vi "save operation binary.vi"(8 "error in":errorcluster, 11 "state cluster":T1) -> (0 "error out":errorcluster, 3 "state out":T1)   [LabVIEW 2013, in "RT Temperature Controller.lvlib"]
uses:
  RT Temperature Controller.lvlib
  Controls/StateCluster.ctl
  <vilib>/NI/Tag Bus Data Framework/Configuration Editor/Classes/SystemConfigRepo/SystemConfigRepo.lvclass
  <vilib>/CEF_TreeControl/Node/NodeRef.ctl
  <vilib>/CEF_TreeControl/Node/NISE_CEF_Node.lvclass
  <vilib>/CEF_TreeControl/Node/UserEventRef.ctl
  <vilib>/CEF_TreeControl/Controls/EventCluster.ctl
  SplashScreen/splash screen.ctl
  SplashScreen/notifier data.ctl
  <vilib>/NI/Tag Bus Data Framework/Configuration Editor/Classes/SystemConfigRepo/SystemConfigRepo.lvclass/SystemConfigRepo.ctl
  <vilib>/CEF_TreeControl/NISE_CEF_TreeControl.lvlib
  SplashScreen/splash screen.lvlib
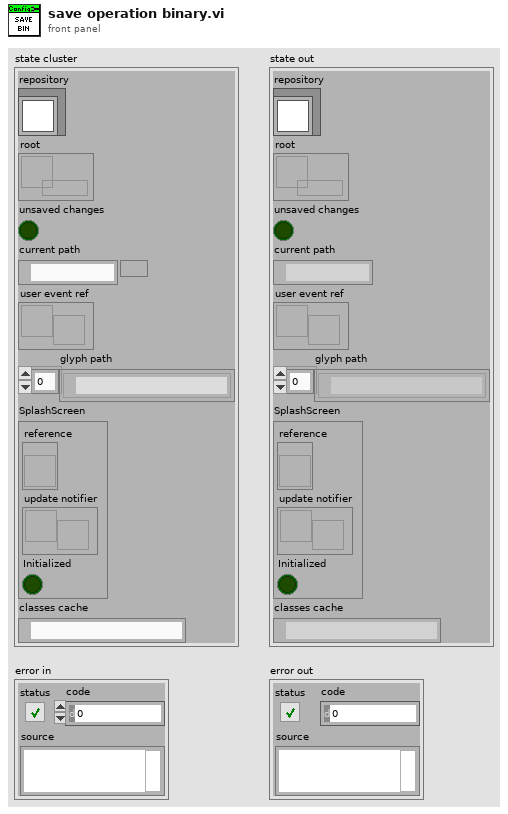
[diagram p1: front panel]
types:
  T1 = typedef "RT Temperature Controller.lvlib/StateCluster.ctl" = cluster{"repository":refnum<class "SystemConfigRepo.lvclass">, "root":T2, "unsaved changes":bool, "current path":path, "user event ref":T3, "glyph path":path[], "SplashScreen":T4, "classes cache":path}
  T2 = typedef "NISE_CEF_Node.lvclass/NodeRef.ctl" = refnum<data-value>
  T3 = typedef "NISE_CEF_Node.lvclass/UserEventRef.ctl" = refnum<user-event>
  T4 = typedef "RT Temperature Controller.lvlib/splash screen.lvlib/splash screen.ctl" = cluster{"reference":refnum<vi>, "update notifier":refnum<notifier>, "Initialized":bool}
  T5 = enum16{"open", "replace", "create", "open or create", "replace or create", "replace or create with confirmation"}
  T6 = typedef "PLConfigurationSerializer.lvlib/systems cluster.ctl" = cluster{"System Configuration":refnum<class "PL_System Configuration.lvclass">, "targets":T7[]}
  T7 = typedef "PLConfigurationSerializer.lvlib/targets cluster.ctl" = cluster{"Target Configuration":refnum<class "PL_Target Configuration.lvclass">, "engines":T8[]}
  T8 = typedef "PLConfigurationSerializer.lvlib/engines cluster.ctl" = cluster{"engine configuration":refnum<class "engine configuration.lvclass">, "modules":refnum<class "TBM module configuration.lvclass">[]}
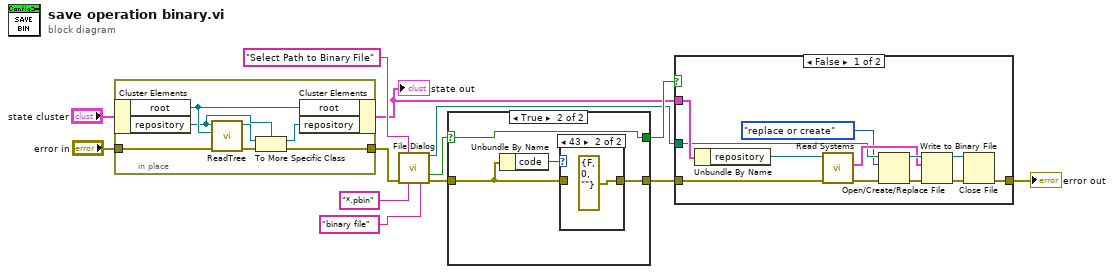
[diagram p0: block diagram]
diagram:
  n1 = in-place {
    in-place-border: "error in" -> [w20]
    in-place-border: [w17] -> w13
    n2 = in-place-cluster #1("state cluster") -> ("root"=w19:T2, "repository"=w15:refnum<class "SystemConfigRepo.lvclass">)
    n3 = call-dynamic "ReadTree.vi"("error in"=w20, "root"=w19, "SystemConfigRepo in"=w15) -> ("error out"=w18:errorcluster, "repository out"=w16:refnum<class "NISE_CEF_Repository.lvclass">)  [unwired: 7 in]
    n4 = To More Specific Class(target class=w15, reference=w16, error in=w18) -> (specific class reference=w14:refnum<class "SystemConfigRepo.lvclass">, error out=w17:errorcluster)
    n5 = in-place-cluster #1("root"=w19, "repository"=w14) -> (w1:T1)
  }
  "state out" <- w1
  n6 = call "File Dialog"("prompt"="Select Path to Binary File" ("Prompt"), "error in"=w13, "pattern (all files)"="*.pbin" ("pattern"), "pattern label"="binary file") -> ("selected path"=w8:path, "cancelled"=w3:bool, "error out"=w2:errorcluster)  [unwired: 8 in, 1 out]
  n7 = case shown="True" w3 {
    selector: w3 -> [w21 w23]
    tunnel: w2 -> [w22 w25]
    tunnel: [w22 w24] -> w7
    tunnel: [w21 w23] -> w9
    frame False {
    }
    frame True {
      n8 = Unbundle By Name(w25) -> ("code"=w26:i32)
      n9 = case shown="43" w26 {
        tunnel: w25 -> [w27 _]
        tunnel: [w27 errorcluster {"status"=FALSE, "code"=0, "source"=""} ("error out")] -> w24
        frame Default {
        }
        frame 43 {
        }
      }
    }
  }
  n10 = case shown="False" w9 {
    tunnel: w1 -> [w40 _]
    tunnel: w7 -> [w38 w41]
    tunnel: [w36 w41] -> w12
    tunnel: w8 -> [w30 _]
    frame False {
      n11 = Unbundle By Name(w40) -> ("repository"=w39:refnum<class "SystemConfigRepo.lvclass">)
      n12 = call <vilib>:"Read Systems.vi"("error in"=w38, "SystemConfigRepo in"=w39) -> ("error out"=w31:errorcluster, "system"=w32:T6)  [unwired: 7 in, 1 out]
      n13 = Open/Create/Replace File(file path (use dialog)=w30, error in=w31, operation (0:open)=T5."replace or create") -> (refnum out=w34:refnum<file>, error out=w33:errorcluster)  [unwired: 3 in, 1 out]
      n14 = Write to Binary File(file (use dialog)=w34, data=w32, error in=w33) -> (refnum out=w35:refnum<file>, error out=w37:errorcluster)  [unwired: 3 in, 1 out]
      n15 = Close File(refnum=w35, error in=w37) -> (error out=w36:errorcluster)  [unwired: 1 out]
    }
    frame True {
    }
  }
  "error out" <- w12
